vi "DEV All Nodes Issue 70.vi"() -> ()   [LabVIEW 2017, in "JSONtext.lvlib"]
uses:
  JSONtext.lvlib
panel:
  in  "Tree":string(tree)
  out "<JSON>":string[](array[string]) caption="<JSON>Items"
  out "$Paths":string[](array[string])
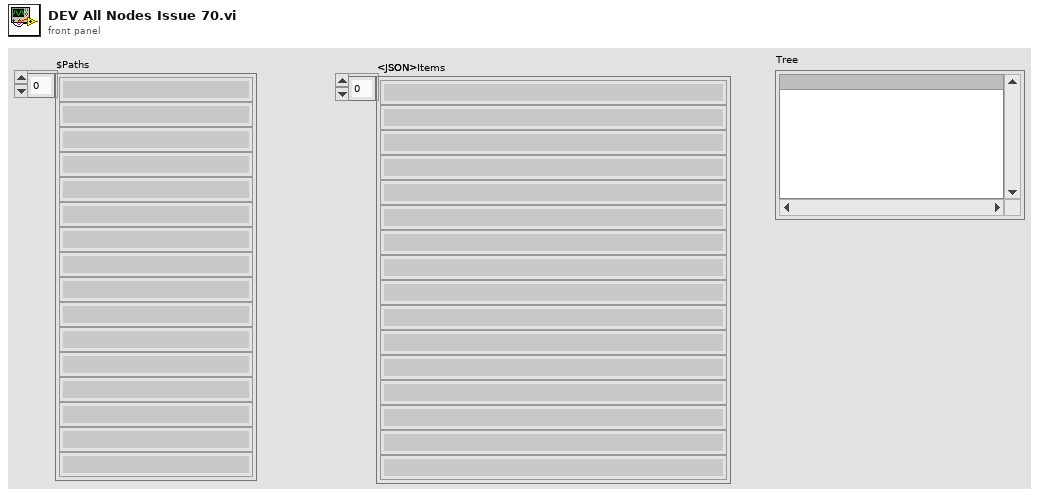
[diagram p1: front panel]
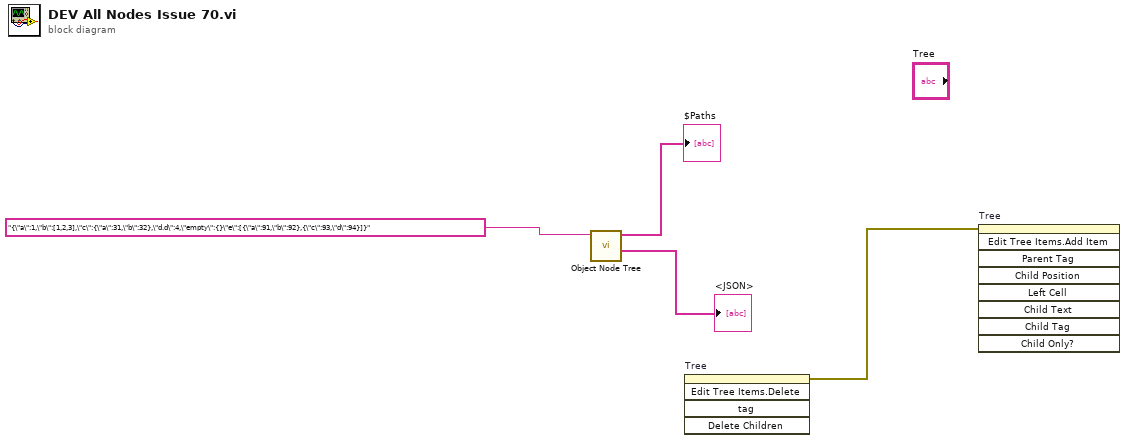
[diagram p0: block diagram]
diagram:
  n1 = call "Object Node Tree.vi"("JSON"="{\"a\":1,\"b\":[1,2,3],\"c\":{\"a\":31,\"b\":32},\"d.d\":4,\"empty\":{}\"e\":[{\"a\":91,\"b\":92},{\"c\":93,\"d\":94}]}") -> ("<JSON>"=→"<JSON>":string[], "$Paths"=→"$Paths":string[])  [unwired: 8 in, 1 out]
  n2 = invoke on="Tree" class="Tree (strict)" method="Edit Tree Items.Delete"() -> (error out=w1:errorcluster)  [unwired: 5 in, 4 out]
  n3 = invoke on="Tree" class="Tree (strict)" method="Edit Tree Items.Add Item"(error in=w1) -> ()  [unwired: 8 in, 9 out]
